vi "GasSensor.vi"() -> ()   [LabVIEW 2022 SP3]
uses:
  <vilib>/DAQmx/read.llb/DAQmx Read (Analog DBL 1Chan 1Samp).vi
  <vilib>/DAQmx/create/channels.llb/DAQmx Create Channel (AI-Voltage-Basic).vi
  <vilib>/DAQmx/miscellaneous.llb/DAQmx Fill In Error Info.vi
panel:
  out "Gas Detected":bool
  out "Meter":dbl(knob) scale=-1.0..7.0
  in  "stop":bool
  in  "physical channels":tag
  out "Waveform Chart":dbl(graph)
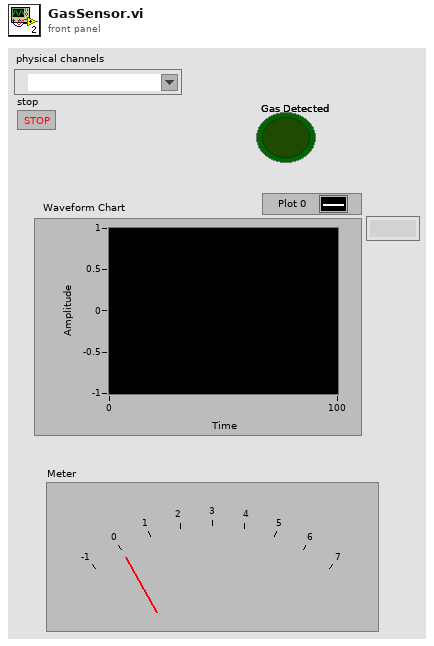
[diagram p1: front panel]
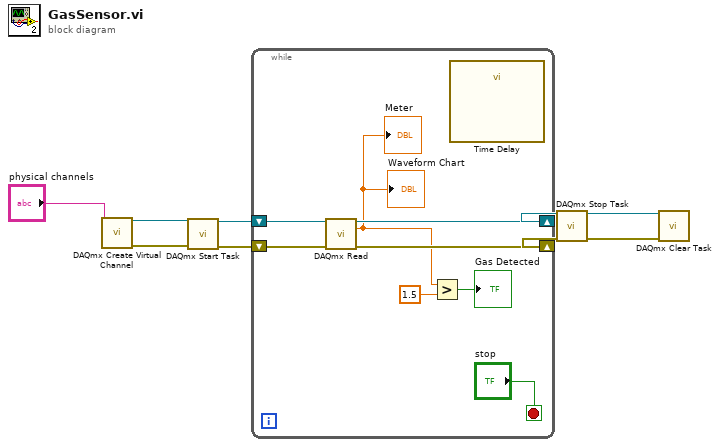
[diagram p0: block diagram]
diagram:
  n1 = call-poly <vilib>:"DAQmx Create Virtual Channel.vi"("physical channels"="physical channels") -> ("task out"=w9:refnum<k21>, "error out"=w6:errorcluster)  [unwired: 13 in]
  n2 = call <vilib>:"DAQmx Start Task.vi"("task/channels in"=w9, "error in"=w6) -> ("task out"=w4:refnum<k21>, "error out"=w3:errorcluster)  [unwired: 12 in]
  n3 = while {
    shift-right: [w15] -> w2
    shift-left: w4 -> [w17]
    shift-right: [w14] -> w1
    shift-left: w3 -> [w16]
    stop <- "stop" stop-if-true
    n4 = call-poly <vilib>:"DAQmx Read.vi"("task/channels in"=w17, "error in"=w16) -> ("task out"=w15:refnum<k21>, "data"=w11:dbl, "error out"=w14:errorcluster)  [unwired: 11 in]
    "Waveform Chart" <- w11
    "Meter" <- w11
    n5 = Greater?(x=w11, y=1.5) -> (0:→"Gas Detected":bool)
    n6 = call "Time Delay"() -> ()  [unwired: 11 in, 1 out]
  }
  n7 = call <vilib>:"DAQmx Stop Task.vi"("task/channels in"=w2, "error in"=w1) -> ("task out"=w8:refnum<k21>, "error out"=w7:errorcluster)  [unwired: 12 in]
  n8 = call <vilib>:"DAQmx Clear Task.vi"("task in"=w8, "error in"=w7) -> ()  [unwired: 13 in, 1 out]
